vi "String.Variant to 2D String.vi"(7 "Ignore Error":bool=TRUE, 8 "Variant":variant) -> (2 "error out":errorcluster, 3 "2DStr":string[][](array[string]))   [LabVIEW 2018]
uses:
  Errors/Error.Error Code List.ctl
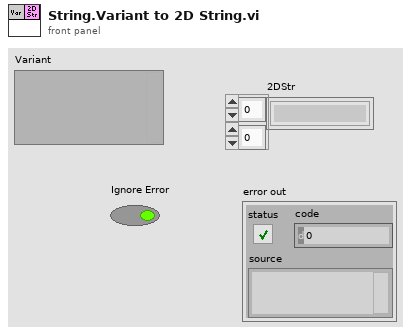
[diagram p1: front panel]
types:
  T1 = typedef "Error.Error Code List.ctl" = i32
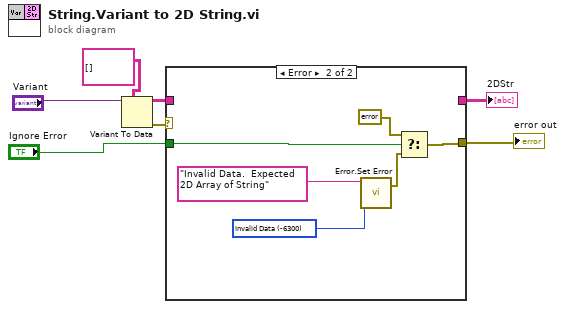
[diagram p0: block diagram]
diagram:
  n1 = Variant To Data(type=string[][] [], Variant="Variant") -> (data=w6:string[][], error out=w5:errorcluster)  [unwired: 1 in]
  n2 = case shown="Error" w5 {
    tunnel: w6 -> [w8 _]
    tunnel: [w8 _] -> w3
    tunnel: "Ignore Error" -> [_ w14]
    tunnel: [_ w12] -> w1
    frame No Error {
    }
    frame Error {
      w10 = T1 -6300 items=["No Error"=0, "Abort"=-2, "Misc"=-5000, "Fixture Error"=-5100, "File IO - General"=-5200, "FIle IO - Config Error"=-5201, "Instrument - General"=-5300, "Instrument - Serial Com"=-5301, "Instrument - Camera"=-5302, "Instrument - PS"=-5303, "Instrument - Oscilloscope"=-5304, "Instrument - Function Gen"=-5305, "Instrument - Load"=-5306, "Instrument - Meter"=-5307, "Instrument - Power Control"=-5308, "Instrument - Motion"=-5309, "Instrument - RF"=-5310, "System Exe"=-5400, "Image Processing"=-5500, "Communication"=-5600, "Script - Syntax Error"=-6000, "Script - Invalid Name or Param"=-6100, "Script - Timeout"=-6200, "Invalid Data"=-6300, "FW Update Error"=-6500] ("Std Code")
      n3 = call "Error.Set Error.vi"("Code"=w10, "Desc"="Invalid Data.  Expected 2D Array of String") -> ("error out"=w9:errorcluster)  [unwired: 5 in]
      n4 = Select(t=errorcluster {"status"=FALSE, "code"=0, "source"=""} ("error constant"), s=w14, f=w9) -> (s? t:f=w12:errorcluster)
    }
  }
  "2DStr" <- w3
  "error out" <- w1
